vi "testProcessCmd.vi"(8 "error in (no error)":errorcluster) -> (0 "error out":errorcluster)   [LabVIEW 2018]
doc: "Test the processCmd.vi."
uses:
  src/TcpServer/TcpServer.lvclass
  src/TcpServer/TcpServer.lvclass/TcpServer.ctl
  src/TcpServerBase/TcpServerBase.lvclass/TcpServerBase.ctl
  src/TcpServerBase/typedef/tcpPacketTypeDef.ctl
  src/TcpServerCmd/TcpServerCmd.lvclass
  home/pcortes/github/ts_labview_tcp_json/src/TcpServerBase/TcpServerBase.lvclass
  <vilib>/addons/_JKI Toolkits/Caraya/classes/Assert/Assert Equal Value_Variant.vi
  <vilib>/addons/_JKI Toolkits/Caraya/classes/Test/Test.lvclass
  <vilib>/addons/_JKI Toolkits/Caraya/classes/Assert/Assert.lvclass
  src/TcpServerBase/TcpServerBase.lvclass
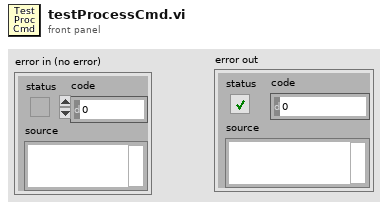
[diagram p1: front panel]
types:
  T1 = typedef "TcpServerBase.lvclass/tcpPacketTypeDef.ctl" = cluster{"packet":string, "firstPacket":bool, "firstConnection":bool}
  T2 = typedef "TcpServer.lvclass/packetConnIDTypeDef.ctl" = cluster{"packet":string, "firstPacket":bool, "firstConnection":bool}
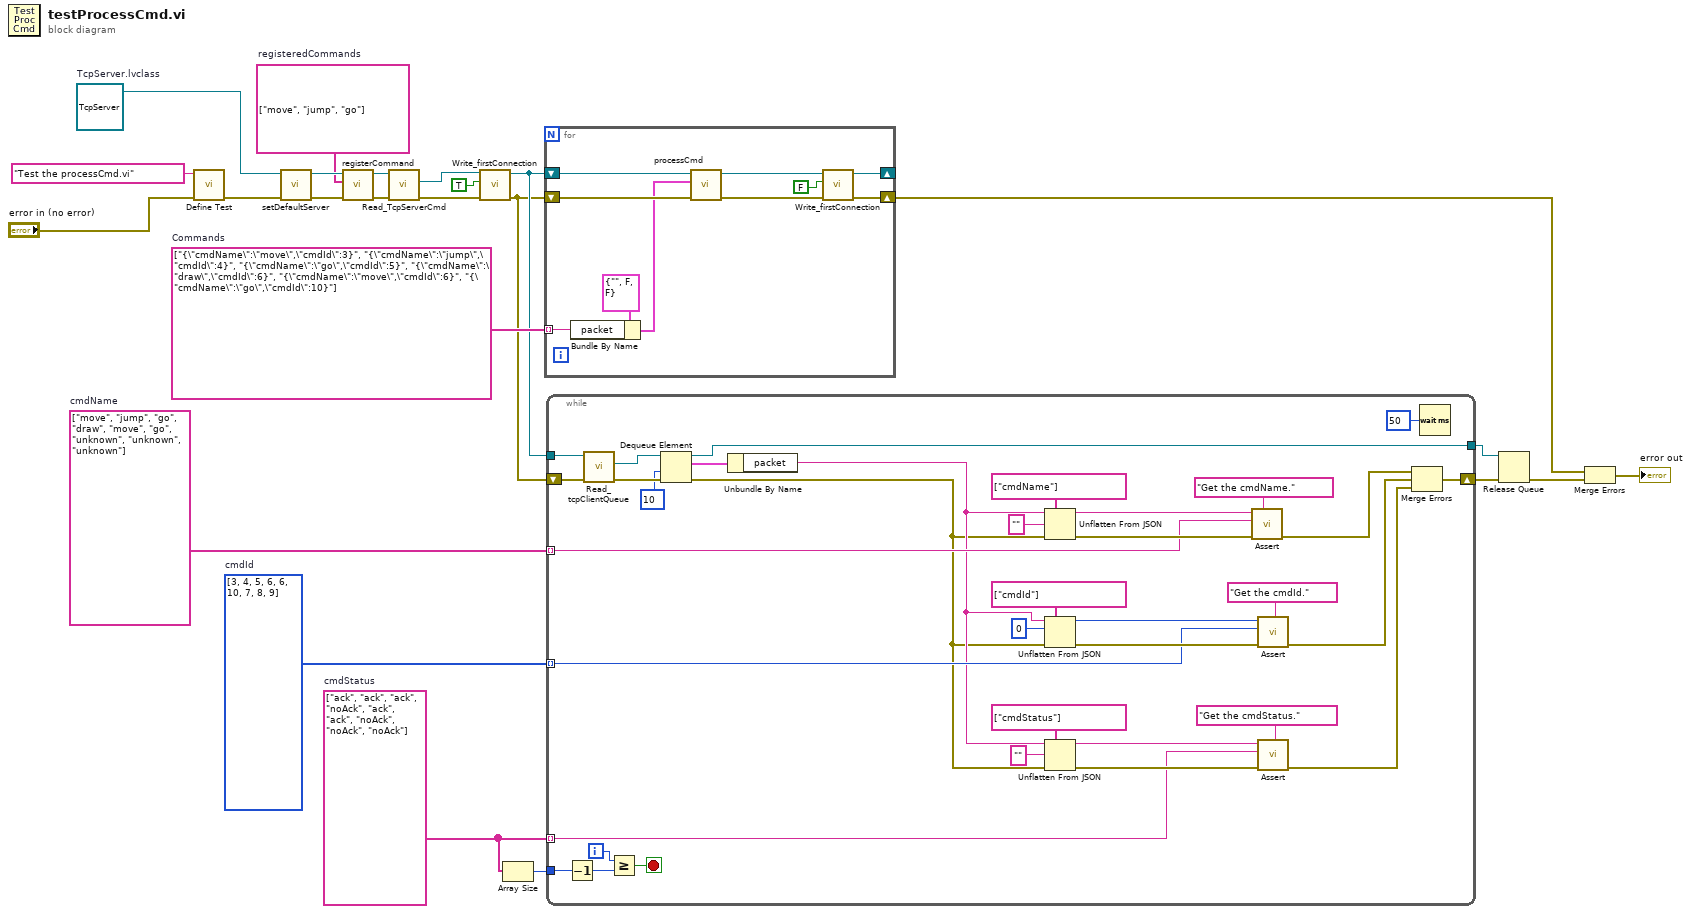
[diagram p0: block diagram]
diagram:
  w9 = string[] ["ack", "ack", "ack", "noAck", "ack", "ack", "noAck", "noAck", "noAck"]  # cmdStatus
  w10 = i32[] [3, 4, 5, 6, 6, 10, 7, 8, 9]  # cmdId
  w11 = string[] ["move", "jump", "go", "draw", "move", "go", "unknown", "unknown", "unknown"]  # cmdName
  w16 = string[] ["{\"cmdName\":\"move\",\"cmdId\":3}", "{\"cmdName\":\"jump\",\"cmdId\":4}", "{\"cmdName\":\"go\",\"cmdId\":5}", "{\"cmdName\":\"draw\",\"cmdId\":6}", "{\"cmdName\":\"move\",\"cmdId\":6}", "{\"cmdName\":\"go\",\"cmdId\":10}"]  # Commands
  w17 = string[] ["move", "jump", "go"]  # registeredCommands
  w21 = refnum<class "TcpServer.lvclass"> refnum  # TcpServer.lvclass
  n1 = call <vilib>:"Define Test.vi"("error in (no error)"="error in (no error)", "Label (VI Title)"="Test the processCmd.vi") -> ("error out"=w23:errorcluster)  [unwired: 9 in]
  n2 = call "setDefaultServer.vi"("error in (no error)"=w23, "TcpServer.lvclass"=w21) -> ("error out"=w19:errorcluster, "tcpServer out"=w18:refnum<class "TcpServer.lvclass">)  [unwired: 8 in]
  n3 = call "registerCommand.vi"("error in (no error)"=w19, "regCommand"=w17, "tcpServer in"=w18) -> ("error out"=w20:errorcluster, "tcpServer out"=w2:refnum<class "TcpServer.lvclass">)  [unwired: 7 in]
  n4 = call "Read_TcpServerCmd.vi"("error in (no error)"=w20, "TcpServer in"=w2) -> ("error out"=w3:errorcluster, "TcpServerCmd.lvclass"=w1:refnum<class "TcpServerCmd.lvclass">)  [unwired: 7 in, 1 out]
  n5 = call "Write_firstConnection.vi"("error in (no error)"=w3, "firstConnection"=TRUE, "TcpServerBase in"=w1) -> ("error out"=w12:errorcluster, "TcpServerBase out"=w13:refnum<class "TcpServerCmd.lvclass">)  [unwired: 7 in]
  n6 = Array Size(array=w9) -> (size(s)=w8:i32)
  n7 = for {
    tunnel: w16 -> [w30] mode=indexing
    shift-right: [w26] -> _
    shift-left: w13 -> [w32]
    shift-right: [w28] -> w7
    shift-left: w12 -> [w34]
    n8 = Bundle By Name(cluster=T1 {"packet"="", "firstPacket"=FALSE, "firstConnection"=FALSE} ("packetConnID"), "packet"=w30) -> (w31:T1)
    n9 = call "processCmd.vi"("error in (no error)"=w34, "tcpPacket"=w31, "tcpServerCmd in"=w32) -> ("error out"=w29:errorcluster, "tcpServerCmd out"=w27:refnum<class "TcpServerCmd.lvclass">)  [unwired: 7 in]
    n10 = call "Write_firstConnection.vi"("error in (no error)"=w29, "firstConnection"=FALSE, "TcpServerBase in"=w27) -> ("error out"=w28:errorcluster, "TcpServerBase out"=w26:refnum<class "TcpServerCmd.lvclass">)  [unwired: 7 in]
  }
  n11 = while {
    tunnel: w13 -> [w67]
    tunnel: w11 -> [w56] mode=indexing
    tunnel: w10 -> [w50] mode=indexing
    tunnel: w9 -> [w49] mode=indexing
    tunnel: w8 -> [w44]
    shift-right: [w38] -> w6
    shift-left: w12 -> [w66]
    tunnel: [w37] -> w4
    i -> [w45]
    stop <- w46 stop-if-true
    n12 = Decrement(x=w44) -> (x-1=w43:i32)
    n13 = call "Read_tcpClientQueue.vi"("error in (no error)"=w66, "TcpServerBase in"=w67) -> ("error out"=w69:errorcluster, "tcpClientQueue"=w68:refnum<queue>)  [unwired: 7 in, 1 out]
    n14 = Greater Or Equal?(x=w45, y=w43) -> (x >= y?=w46:bool)
    n15 = Dequeue Element(queue=w68, timeout in ms (-1)=10, error in (no error)=w69) -> (queue out=w37:refnum<queue>, element=w70:T2, error out=w42:errorcluster)  [unwired: 1 out]
    n16 = Unbundle By Name(w70) -> ("packet"=w48:string)
    n17 = Unflatten From JSON(path=string[] ["cmdName"], JSON string=w48, type and defaults="" ("packet"), error in (no error)=w42) -> (value=w63:string, error out=w60:errorcluster)  [unwired: 3 in]
    n18 = Unflatten From JSON(path=string[] ["cmdId"], JSON string=w48, type and defaults=0, error in (no error)=w42) -> (value=w64:i32, error out=w59:errorcluster)  [unwired: 3 in]
    n19 = Unflatten From JSON(path=string[] ["cmdStatus"], JSON string=w48, type and defaults="" ("packet"), error in (no error)=w42) -> (value=w52:string, error out=w54:errorcluster)  [unwired: 3 in]
    n20 = call-poly <vilib>:"Assert.vi"("Label"="Get the cmdName.", "error in (no error)"=w60, "Y"=w56, "X"=w63) -> ("error out"=w41:errorcluster)  [unwired: 7 in]
    n21 = call-poly <vilib>:"Assert.vi"("Label"="Get the cmdId.", "error in (no error)"=w59, "Y"=w50, "X"=w64) -> ("error out"=w40:errorcluster)  [unwired: 7 in]
    n22 = call-poly <vilib>:"Assert.vi"("Label"="Get the cmdStatus.", "error in (no error)"=w54, "Y"=w49, "X"=w52) -> ("error out"=w39:errorcluster)  [unwired: 7 in]
    n23 = Merge Errors(w41, w40, w39) -> (w38:errorcluster)
    n24 = Wait (ms)(milliseconds to wait=u32 50) -> ()  [unwired: 1 out]
  }
  n25 = Release Queue(queue=w4, error in (no error)=w6) -> (error out=w5:errorcluster)  [unwired: 1 in, 2 out]
  n26 = Merge Errors(w7, w5) -> (→"error out":errorcluster)
